vi "cDAQ RH and Temp Convert AI Volt to Measurement.vi"(9 "Test Setup":T2, 10 "Temp Volt":T1, 11 "RH Volt":T1) -> (2 "Temp Mean measurement (F)":dbl, 3 "RH Mean measurement (%)":dbl)   [LabVIEW 2014]
doc: "Used to find RH and temp from Dwyer 576-1"
uses:
  Type Definitions/cDAQ Instrument Sensor.ctl
panel:
  out "Temp Std dev measurement":dbl
  out "RH Std dev measurement":dbl
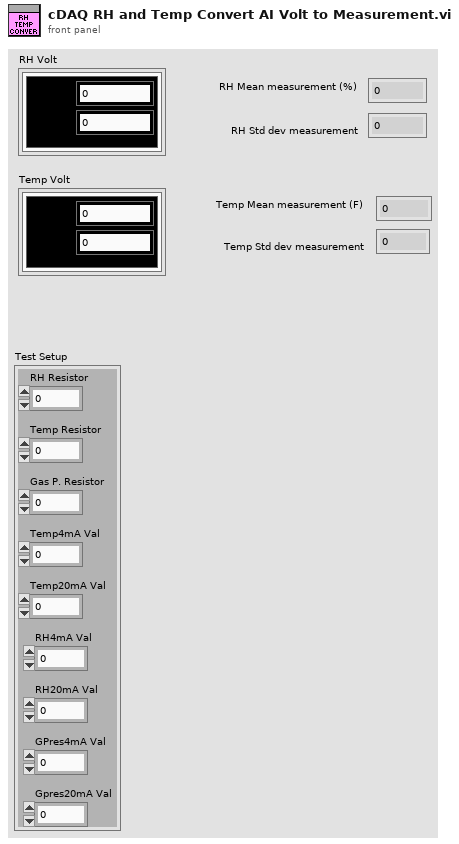
[diagram p1: front panel]
types:
  T1 = typedef "cDAQ Instrument Sensor.ctl" = cluster{"Mean":dbl, " Std":dbl, "Color Box":u32}
  T2 = cluster{"RH Resistor":dbl, "Temp Resistor":dbl, "Gas P. Resistor":dbl, "Temp4mA Val":dbl, "Temp20mA Val":dbl, "RH4mA Val":dbl, "RH20mA Val":dbl, "GPres4mA Val":dbl, "Gpres20mA Val":dbl}
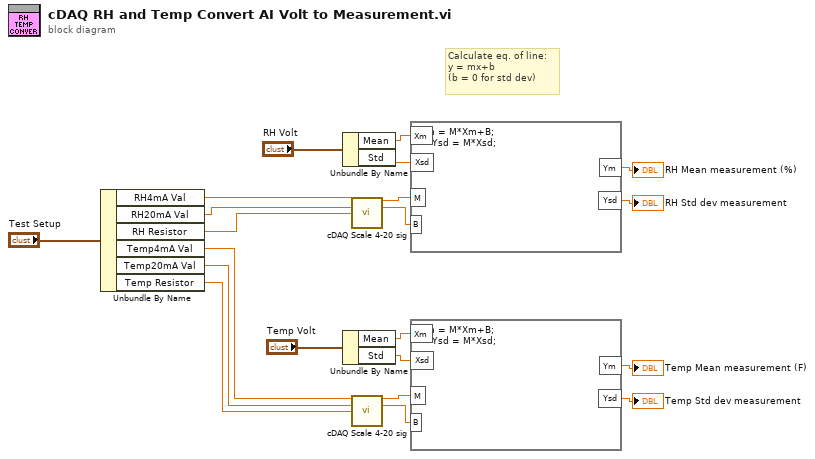
[diagram p0: block diagram]
diagram:
  # "Calculate eq. of line: \ny = mx+b \n(b = 0 for std dev)"
  n1 = Unbundle By Name("Test Setup") -> ("RH4mA Val"=w13:dbl, "RH20mA Val"=w12:dbl, "RH Resistor"=w11:dbl, "Temp4mA Val"=w10:dbl, "Temp20mA Val"=w9:dbl, "Temp Resistor"=w8:dbl)
  n2 = Unbundle By Name("RH Volt") -> ("Mean"=w18:dbl, "Std"=w16:dbl)
  n3 = Unbundle By Name("Temp Volt") -> ("Mean"=w5:dbl, "Std"=w3:dbl)
  n4 = call "cDAQ Scale 4-20 sig.vi"("4 mA y- value"=w13, "20 mA y-value"=w12, "Drop resistor"=w11) -> ("M"=w21:dbl, "B"=w20:dbl)  [unwired: 11 in]
  n5 = call "cDAQ Scale 4-20 sig.vi"("4 mA y- value"=w10, "20 mA y-value"=w9, "Drop resistor"=w8) -> ("M"=w7:dbl, "B"=w6:dbl)  [unwired: 11 in]
  n6 = formula code="Ym = M*Xm+B;\n    Ysd = M*Xsd;"("M"=w21, "B"=w20, "Xm"=w18, "Xsd"=w16) -> ("Ym"=→"RH Mean measurement (%)":dbl, "Ysd"=→"RH Std dev measurement":dbl)
  n7 = formula code="Ym = M*Xm+B;\n    Ysd = M*Xsd;"("M"=w7, "B"=w6, "Xm"=w5, "Xsd"=w3) -> ("Ym"=→"Temp Mean measurement (F)":dbl, "Ysd"=→"Temp Std dev measurement":dbl)
